vi "strober.vi"(11 "input reference":T1={"inner index"=0, "outer index"=0, "array"=[], "value"=TRUE, "count"=0}) -> (0 "new data":bool, 1 "output ticks":i32[](array[numeric]), 3 "output reference":T1)   [LabVIEW 2019]
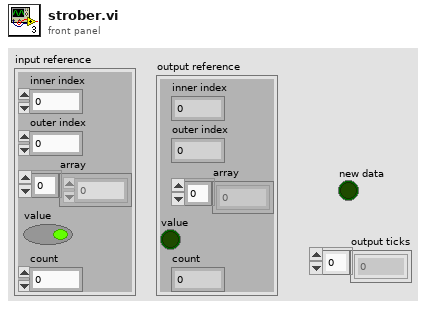
[diagram p1: front panel]
types:
  T1 = cluster{"inner index":i32, "outer index":i32, "array":i32[], "value":bool, "count":i32}
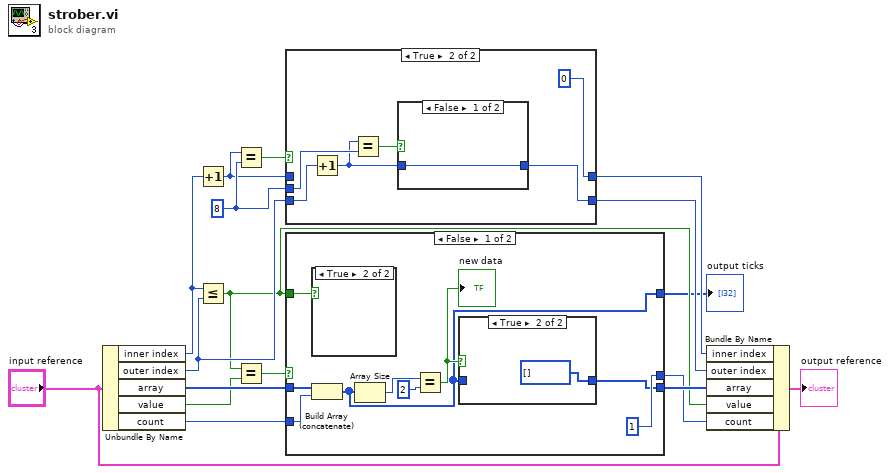
[diagram p0: block diagram]
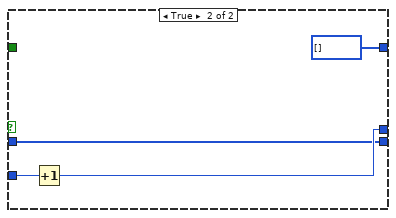
[diagram p4: hidden frame]
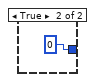
[diagram p6: hidden frame]
diagram:
  w17 = 8
  n1 = Unbundle By Name("input reference") -> ("inner index"=w13:i32, "outer index"=w10:i32, "array"=w12:i32[], "value"=w9:bool, "count"=w11:i32)
  n2 = Increment(x=w13) -> (x+1=w15:i32)
  n3 = Less Or Equal?(x=w13, y=w10) -> (x <= y?=w3:bool)
  n4 = Equal?(x=w15, y=w17) -> (x = y?=w16:bool)
  n5 = Equal?(x=w3, y=w9) -> (x = y?=w14:bool)
  n6 = case shown="True" w16 {
    tunnel: w10 -> [w19 w25]
    tunnel: w17 -> [_ w24]
    tunnel: [w19 w22] -> w6
    tunnel: [w18 0] -> w7
    tunnel: w15 -> [w18 _]
    frame False {
    }
    frame True {
      n7 = Increment(x=w25) -> (x+1=w21:i32)
      n8 = Equal?(x=w21, y=w24) -> (x = y?=w23:bool)
      n9 = case shown="False" w23 {
        tunnel: [w26 0] -> w22
        tunnel: w21 -> [w26 _]
        frame False {
        }
        frame True {
        }
      }
    }
  }
  n10 = case shown="False" w14 {
    tunnel: w11 -> [w28 w42]
    tunnel: [1 w41] -> w4
    tunnel: w3 -> [w35 _]
    tunnel: w12 -> [w34 w40]
    tunnel: [w31 w40] -> w5
    tunnel: [w29 i32[] []] -> w2
    frame False {
      n11 = case shown="True" w35 {
        frame False {
        }
        frame True {
        }
      }
      n12 = Build Array (concatenate)(w34, w28) -> (w29:i32[])
      n13 = Array Size(array=w29) -> (size(s)=w33:i32)
      n14 = Equal?(x=w33, y=2) -> (x = y?=w30:bool)
      "new data" <- w30
      n15 = case shown="True" w30 {
        tunnel: w29 -> [w37 _]
        tunnel: [w37 i32[] []] -> w31
        frame False {
        }
        frame True {
        }
      }
    }
    frame True {
      n16 = Increment(x=w42) -> (x+1=w41:i32)
    }
  }
  "output ticks" <- w2
  n17 = Bundle By Name(cluster="input reference", "inner index"=w7, "outer index"=w6, "array"=w5, "value"=w3, "count"=w4) -> (→"output reference":T1)
